vi "lua_settable.vi"(8 "error in (no error)":errorcluster, 10 "index":i32, 11 "lua_state_p":u64) -> (0 "error out":errorcluster, 3 "lua_state_p out":u64)   [LabVIEW 2020, in "lua.dll.lvlib"]
doc: "Does the equivalent to t[k] = v, where t is the value at the given valid index, v is the value at the top of the stack, and k is the value just below the top.\n\nThis function pops both the key and the value from the stack. As in Lua, this function may trigger a metamethod for the \"newindex\" event (see §2.8)."
uses:
  lua.dll.lvlib
  lua54.dll
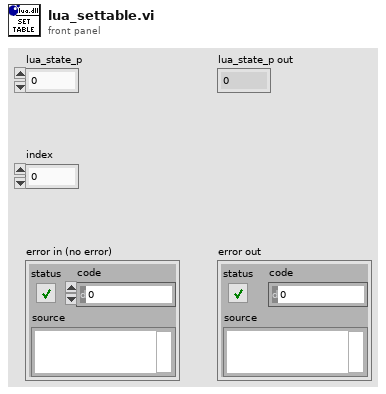
[diagram p1: front panel]
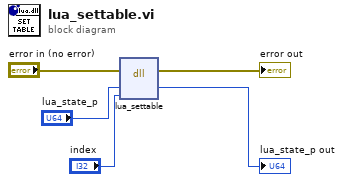
[diagram p0: block diagram]
diagram:
  n1 = dll-call lib="C:/Users/Nicholas Folse/Documents/workspace/github-tauterra.llc/Lua for LabVIEW/lib/lua.dll/lua54**.*" fn="lua_settable"(error in="error in (no error)", "lua_state_p"="lua_state_p", "index"="index") -> (error out=→"error out":errorcluster, "lua_state_p"=→"lua_state_p out":u64)  [unwired: 4 in, 1 out]
